vi "HEWH Read Settings.vi"(0 "Tool Base Path":path, 5 "Error In":errorcluster, 6 "Debug":bool) -> (12 "Intellifaucet Type":string, 14 "K-Factor (Flow)":dbl, 15 "K-Factor (Temperature)":dbl, 16 "Power Analyzer":T2, 17 "Station":string, 18 "LV Program":T1, 19 "Error Out":errorcluster)   [LabVIEW 2016]
uses:
  Utility/Type Definitions/UTILITY Power Analyzer.ctl
  Utility/Save File/File Setup (Public)/Type Definition/Save File DOE LabView Program.ctl
  <vilib>/Utility/error.llb/whitespace.ctl
  <vilib>/Utility/file.llb/Write To Spreadsheet File (string).vi
  <vilib>/Utility/file.llb/Read From Spreadsheet File (string).vi
  Utility/Save File/File Setup.lvlib
panel:
  out "file or folder exists?":bool
  out "RLT?":string
  out "Power Analyzer":string
  out "all rows":string[][](array[string])
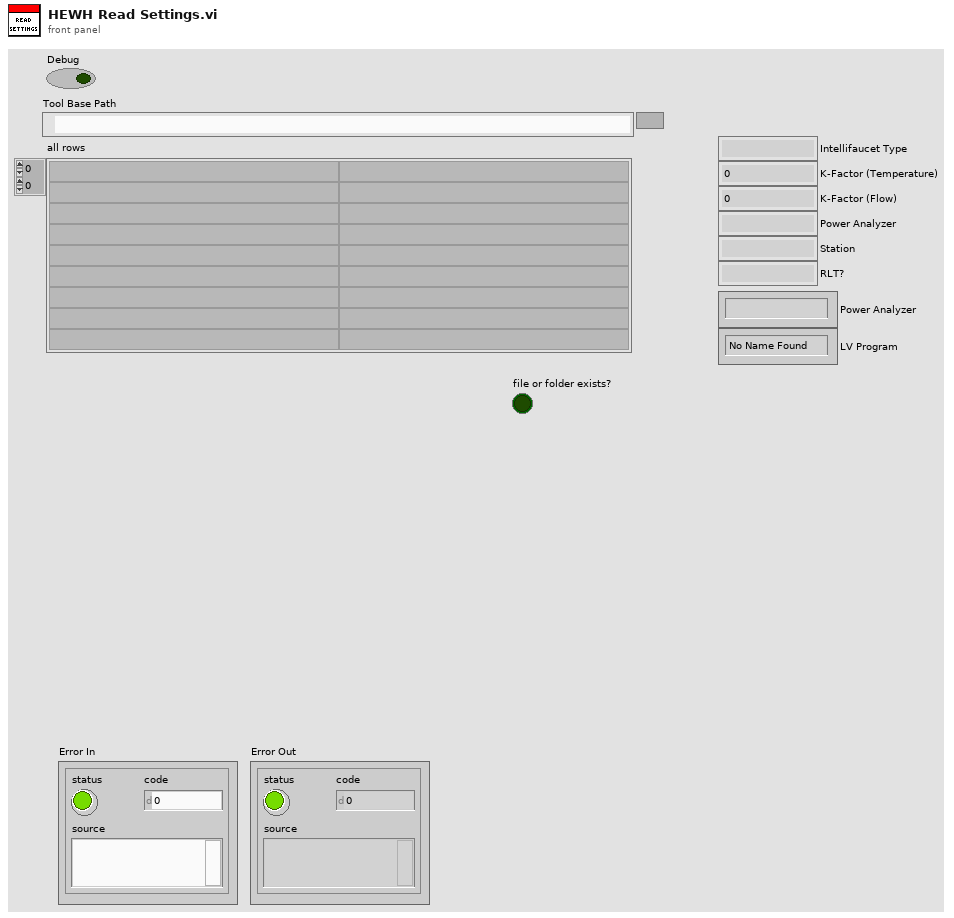
[diagram p1: front panel]
types:
  T1 = typedef "File Setup.lvlib/Save File DOE LabView Program.ctl" = enum16{"No Name Found", "DOE Stand", "Dishwasher Kitchen", "Portable Stand", "HEWH", "Dryer", "Dryer WILT", "HCC", "PRAT", "HEWH RLT", "Refrigeration"}
  T2 = typedef "UTILITY Power Analyzer.ctl" = enum16{"", "APLUS", "WT210", "WT500", "WT300", "OSI", "Debug", "WT230", "WT300_1", "WT300_2"}
  T3 = typedef "whitespace.ctl" = u16
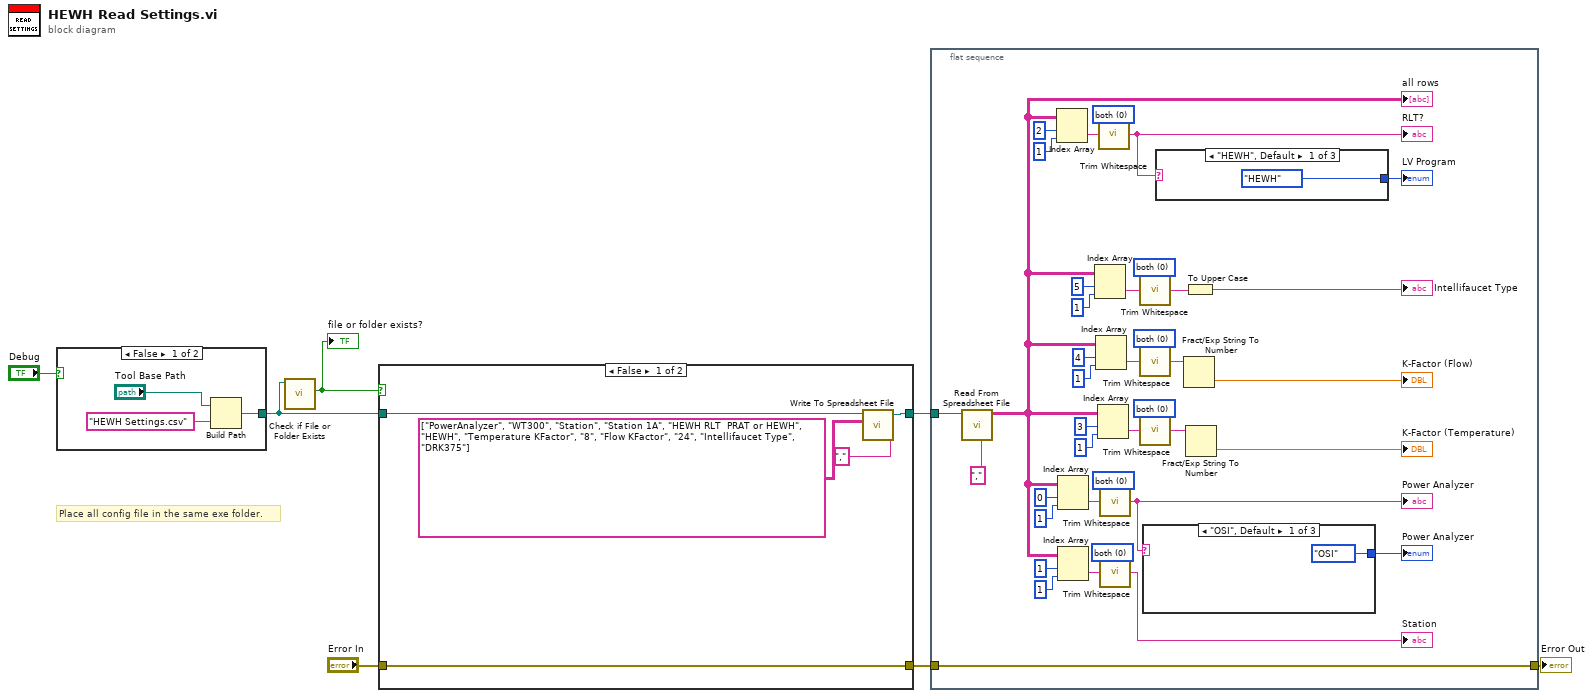
[diagram p0: block diagram]
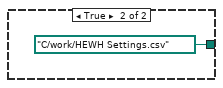
[diagram p2: hidden frame]
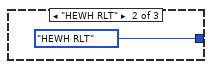
[diagram p3: hidden frame]
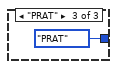
[diagram p4: hidden frame]
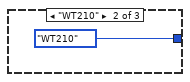
[diagram p5: hidden frame]
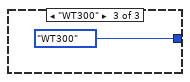
[diagram p6: hidden frame]
diagram:
  # "Place all config file in the same exe folder."
  n1 = case shown="False" "Debug" {
    tunnel: [w8 path "C:/work/HEWH Settings.csv" ("HEWH Settings")] -> w2
    frame False {
      n2 = Build Path(base path="Tool Base Path", name or relative path="HEWH Settings.csv") -> (appended path=w8:path)
    }
    frame True {
    }
  }
  n3 = call <vilib>:"Check if File or Folder Exists.vi"("path"=w2) -> ("file or folder exists?"=w7:bool)  [unwired: 8 in, 2 out]
  "file or folder exists?" <- w7
  n4 = case shown="False" w7 {
    tunnel: w2 -> [w16 w17]
    tunnel: "Error In" -> [w13 w18]
    tunnel: [w13 w18] -> w5
    tunnel: [w12 w17] -> w3
    frame False {
      n5 = call-poly <vilib>:"Write To Spreadsheet File.vi"("delimiter (\\t)"="," ("delimiter (\\t)"), "2D data"=string[][] [["PowerAnalyzer", "WT300"], ["Station", "Station 1A"], ["HEWH RLT  PRAT or HEWH", "HEWH"], ["Temperature KFactor", "8"], ["Flow KFactor", "24"], ["Intellifaucet Type", "DRK375"]] ("all rows 2"), "file path (dialog if empty)"=w16) -> ("new file path (Not A Path if cancelled)"=w12:path)  [unwired: 5 in]
    }
    frame True {
    }
  }
  n6 = flat-sequence {
    tunnel: w3 -> [w37]
    tunnel: w5 -> [w36]
    tunnel: [w36] -> w4
    frame #0 {
      w25 = T3 0 items=["both", "start of string", "end of string"] ("location (both)")
      w27 = T3 0 items=["both", "start of string", "end of string"] ("location (both)")
      w28 = T3 0 items=["both", "start of string", "end of string"] ("location (both)")
      w29 = T3 0 items=["both", "start of string", "end of string"] ("location (both)")
      w30 = T3 0 items=["both", "start of string", "end of string"] ("location (both)")
      w31 = T3 0 items=["both", "start of string", "end of string"] ("location (both)")
      n7 = call-poly <vilib>:"Read From Spreadsheet File.vi"("delimiter (\\t)"="," ("delimiter (\\t)"), "file path (dialog if empty)"=w37) -> ("all rows"=w21:string[][])  [unwired: 5 in, 4 out]
      "all rows" <- w21
      n8 = Index Array(array=w21, index (row)=2 ("disabled index (row)"), index (col)=1 ("disabled index (col)")) -> (element=w48:string)
      n9 = Index Array(array=w21, index (row)=0 ("disabled index (row)"), index (col)=1 ("disabled index (col)")) -> (element=w54:string)
      n10 = Index Array(array=w21, index (row)=1 ("disabled index (row)"), index (col)=1 ("disabled index (col)")) -> (element=w53:string)
      n11 = Index Array(array=w21, index (row)=5 ("disabled index (row)"), index (col)=1 ("disabled index (col)")) -> (element=w24:string)
      n12 = Index Array(array=w21, index (row)=4 ("disabled index (row)"), index (col)=1 ("disabled index (col)")) -> (element=w32:string)
      n13 = Index Array(array=w21, index (row)=3 ("disabled index (row)"), index (col)=1 ("disabled index (col)")) -> (element=w46:string)
      n14 = call <vilib>:"Trim Whitespace.vi"("string"=w48, "location (both)"=w30) -> ("trimmed string"=w39:string)
      "RLT?" <- w39
      n15 = call <vilib>:"Trim Whitespace.vi"("string"=w54, "location (both)"=w28) -> ("trimmed string"=w41:string)
      "Power Analyzer" <- w41
      n16 = call <vilib>:"Trim Whitespace.vi"("string"=w53, "location (both)"=w27) -> ("trimmed string"=→"Station":string)
      n17 = call <vilib>:"Trim Whitespace.vi"("string"=w24, "location (both)"=w25) -> ("trimmed string"=w20:string)
      n18 = call <vilib>:"Trim Whitespace.vi"("string"=w32, "location (both)"=w31) -> ("trimmed string"=w35:string)
      n19 = call <vilib>:"Trim Whitespace.vi"("string"=w46, "location (both)"=w29) -> ("trimmed string"=w43:string)
      n20 = case shown="\"OSI\", Default" w41 {
        tunnel: [UTILITY_Power_Analyzer."OSI" ("Power Analyzer") UTILITY_Power_Analyzer."WT210" ("Power Analyzer") UTILITY_Power_Analyzer."WT300" ("Power Analyzer")] -> w40
        frame "OSI", Default {
        }
        frame "WT210" {
        }
        frame "WT300" {
        }
      }
      "Power Analyzer" <- w40
      n21 = case shown="\"HEWH\", Default" w39 {
        tunnel: [Save_File_DOE_LabView_Program."HEWH" ("LV Program") Save_File_DOE_LabView_Program."HEWH RLT" ("LV Program") Save_File_DOE_LabView_Program."PRAT" ("LV Program")] -> w38
        frame "HEWH", Default {
        }
        frame "HEWH RLT" {
        }
        frame "PRAT" {
        }
      }
      "LV Program" <- w38
      n22 = Fract/Exp String To Number(string=w35) -> (number=→"K-Factor (Flow)":dbl)  [unwired: 3 in, 1 out]
      n23 = To Upper Case(1:w20) -> (0:→"Intellifaucet Type":string)
      n24 = Fract/Exp String To Number(string=w43) -> (number=→"K-Factor (Temperature)":dbl)  [unwired: 3 in, 1 out]
    }
  }
  "Error Out" <- w4
